vi "Write Data Queue.vi"(8 "error in (no error)":errorcluster, 10 "Data Queue":refnum<queue>, 11 "Analog Reader in":refnum<class "Analog Reader.lvclass">) -> (0 "error out":errorcluster, 3 "Analog Reader out":refnum<class "Analog Reader.lvclass">)   [LabVIEW 2024, in "DAQmx Actor.lvlib" / "Analog Reader.lvclass"]
uses:
  Analog Reader.lvclass
  Analog Reader.lvclass/Analog Reader.ctl
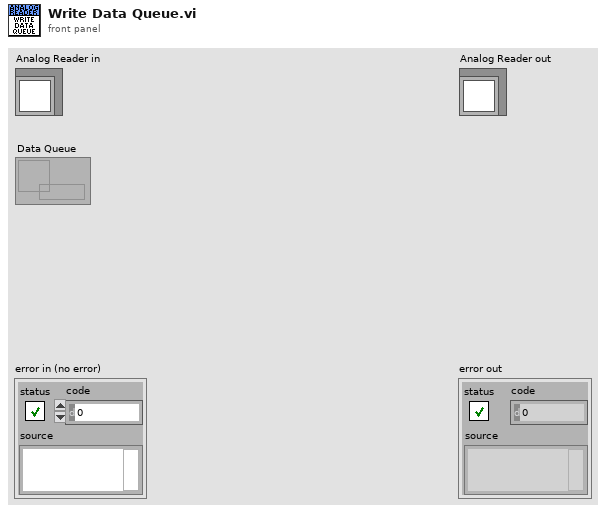
[diagram p1: front panel]
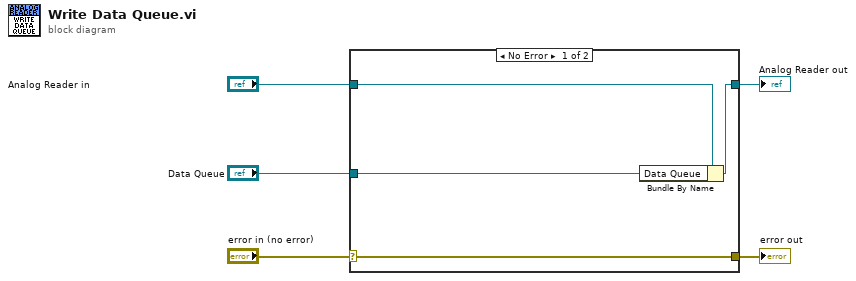
[diagram p0: block diagram]
diagram:
  n1 = case shown="No Error" "error in (no error)" {
    selector: "error in (no error)" -> [w9 w10]
    tunnel: [w9 w10] -> w4
    tunnel: [w7 w11] -> w2
    tunnel: "Analog Reader in" -> [w8 w11]
    tunnel: "Data Queue" -> [w6 _]
    frame No Error {
      n2 = Bundle By Name(cluster=w8, "Data Queue"=w6) -> (w7:refnum<class "Analog Reader.lvclass">)
    }
    frame Error {
    }
  }
  "error out" <- w4
  "Analog Reader out" <- w2
